vi "Global.vi"() -> ()   [LabVIEW 2024]
panel:
  in  "Mode":string
  in  "Open %":dbl
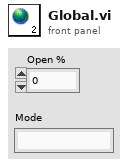
[diagram p1: front panel]
diagram:
